vi "Convert_StringToU8.vi"(9 "node text":string) -> (1 "Numeric":u8)   [LabVIEW 2010, in "Pansino_XML_Read.lvlib"]
uses:
  Pansino_XML_Read.lvlib
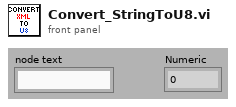
[diagram p1: front panel]
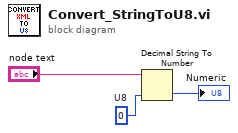
[diagram p0: block diagram]
diagram:
  w1 = u8 0  # U8
  n1 = Decimal String To Number(string="node text", default (0L)=w1) -> (number=→"Numeric":u8)  [unwired: 1 in, 1 out]
